vi "Redraw full indicator.vi"(8 "error in (no error)":errorcluster, 11 "D_Datagrid in":refnum<class "D_Datagrid.lvclass">) -> (0 "error out":errorcluster, 3 "D_Datagrid out":refnum<class "D_Datagrid.lvclass">)   [LabVIEW 2023, in "D Datagrid Library.lvlib" / "D_Datagrid.lvclass"]
doc: "Redraws the control to show the current DataElements value. If \"Auto Update Indicator\" is True, this is called automatically when writing DataElements. Otherwise, you should call this manually when you want to update the indicator."
uses:
  D_Datagrid.lvclass
  C:/Program Files/National Instruments/LabVIEW 2023/vi.lib/QSI/QControls/QControl Classes/Control/Control.lvclass
  C:/Program Files/National Instruments/LabVIEW 2023/vi.lib/QSI/QControls/QControl Classes/Table/Table.lvclass
  D_Datagrid.lvclass/D_Datagrid.ctl
  DatagridElement/DatagridElement.lvclass/DatagridElement.ctl
  <vilib>/Utility/miscctls.llb/LVRowAndColumnTypeDef.ctl
  DatagridElement/Read Cell font.vi
  DatagridElement/Read Text Alpha.vi
  DatagridElement/Read Enabled state.vi
  Read DataElements.vi
  <vilib>/Utility/colorconv.llb/Color to RGB.vi
  <vilib>/Utility/colorconv.llb/RGB to Color.vi
  DatagridElement/DatagridElement.lvclass
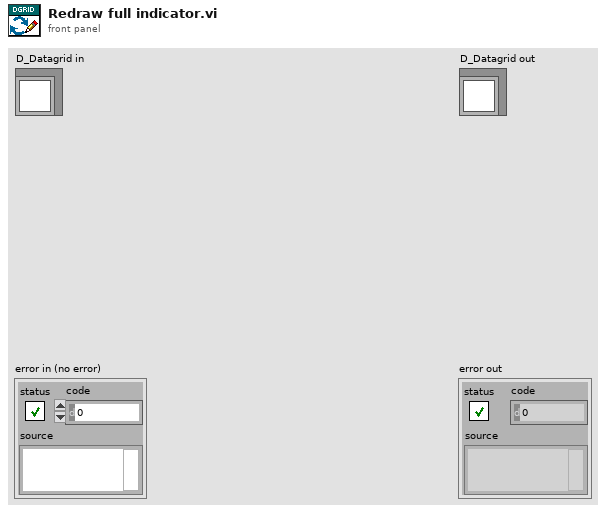
[diagram p1: front panel]
types:
  T1 = typedef "LVFontTypeDef.ctl" = cluster{"Font Name":string, "Size":u16, "Bold":bool, "Italic":bool, "Underline":bool, "Strikeout":bool, "Color":u32}
  T2 = enum8{"Enabled", "Disabled", "Disabled and Grayed Out"}
  T3 = cluster{"Accessors:Cell font":T1, "Accessors:Text Alpha":dbl, "Accessors:Enabled state":enum8{"Enabled", "Disabled", "Disabled and Grayed Out"}, i32, i32}
  T4 = typedef "LVRowAndColumnTypeDef.ctl" = cluster{"Row":i32, "Column":i32}
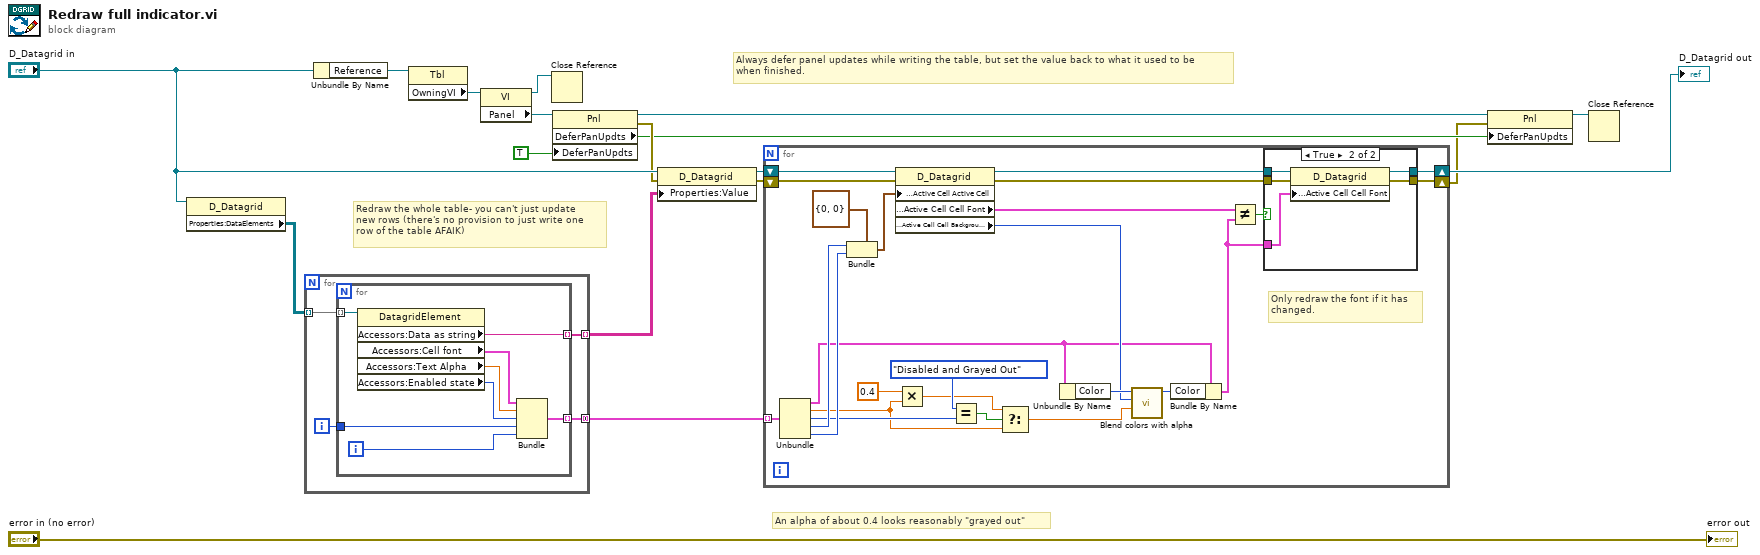
[diagram p0: block diagram]
diagram:
  # "An alpha of about 0.4 looks reasonably \"grayed out\""
  # "Redraw the whole table- you can't just update\nnew rows (there's no provision to just write one\nrow of the table AFAIK)"
  # "Always defer panel updates while writing the table, but set the value back to what it used to be\nwhen finished."
  n1 = property class="D_Datagrid"(reference="D_Datagrid in") -> ("Properties:DataElements"=w3:refnum<class "DatagridElement.lvclass">[][])  [unwired: 1 in, 2 out]
  n2 = for {
    tunnel: w3 -> [w22] mode=indexing
    tunnel: [w21] -> w15 mode=indexing
    tunnel: [w19] -> w13 mode=concatenating
    i -> [w20]
    n3 = for {
      tunnel: w22 -> [w30] mode=indexing
      tunnel: [w29] -> w21 mode=indexing
      tunnel: w20 -> [w28]
      tunnel: [w26] -> w19 mode=indexing
      i -> [w27]
      n4 = property class="DatagridElement"(reference=w30) -> ("Accessors:Data as string"=w29:string, "Accessors:Cell font"=w24:T1, "Accessors:Text Alpha"=w23:dbl, "Accessors:Enabled state"=w25:T2)  [unwired: 1 in, 2 out]
      n5 = Bundle("Accessors:Cell font"=w24, "Accessors:Text Alpha"=w23, "Accessors:Enabled state"=w25, w28, w27) -> (w26:T3)  [unwired: 1 in]
    }
  }
  n6 = Unbundle By Name("D_Datagrid in") -> ("Reference"=w12:refnum<vi>)
  n7 = property class="Tbl"(reference=w12) -> ("OwningVI"=w11:refnum<vi>)  [unwired: 1 in, 2 out]
  n8 = property class="VI"(reference=w11) -> (reference out=w9:refnum<vi>, "Panel"=w5:refnum<vi>)  [unwired: 1 in, 1 out]
  n9 = Close Reference(reference=w9) -> ()  [unwired: 1 in, 1 out]
  n10 = property class="Pnl"(reference=w5, "DeferPanUpdts"=TRUE ("Defer Panel Updates")) -> (reference out=w8:refnum<vi>, error out=w10:errorcluster, "DeferPanUpdts"=w4:bool)  [unwired: 1 in]
  n11 = property class="D_Datagrid"(reference="D_Datagrid in", error in=w10, "Properties:Value"=w15) -> (reference out=w14:refnum<class "D_Datagrid.lvclass">, error out=w2:errorcluster)
  n12 = for {
    shift-right: [w49] -> w16
    shift-left: w14 -> [w55]
    tunnel: w13 -> [w54] mode=indexing
    shift-right: [w44] -> w1
    shift-left: w2 -> [w46]
    # "Only redraw the font if it has\nchanged."
    n13 = Unbundle(w54) -> ("Accessors:Cell font"=w33:T1, "Accessors:Text Alpha"=w37:dbl, "Accessors:Enabled state"=w39:T2, w43:i32, w42:i32)
    n14 = Bundle(cluster=T4 {"Row"=0, "Column"=0} ("Active Cell:Active Cell"), "Row"=w43, "Column"=w42) -> (w51:T4)
    n15 = property class="D_Datagrid"(reference=w55, error in=w46, "Properties:Active Cell Active Cell"=w51) -> (reference out=w50:refnum<class "D_Datagrid.lvclass">, error out=w45:errorcluster, "Properties:Active Cell Cell Font"=w48:T1, "Properties:Active Cell Cell Background Color"=w35:u32)
    n16 = Multiply(x=0.4 ("y"), y=w37) -> (x*y=w38:dbl)
    n17 = Equal?(x=T2."Disabled and Grayed Out" ("Accessors:Enabled state"), y=w39) -> (x = y?=w40:bool)
    n18 = Select(t=w38, s=w40, f=w37) -> (s? t:f=w34:dbl)
    n19 = Unbundle By Name(w33) -> ("Color"=w36:u32)
    n20 = call "Blend colors with alpha.vi"("Top alpha"=w34, "Bottom color"=w35, "Top color"=w36) -> ("Result color"=w32:u32)  [unwired: 7 in, 1 out]
    n21 = Bundle By Name(cluster=w33, "Color"=w32) -> (w31:T1)
    n22 = Not Equal?(x=w48, y=w31) -> (x != y?=w47:bool)
    n23 = case shown="True" w47 {
      tunnel: w50 -> [w57 w62]
      tunnel: [w57 w61] -> w49
      tunnel: w45 -> [w56 w60]
      tunnel: [w56 w59] -> w44
      tunnel: w31 -> [_ w58]
      frame False {
      }
      frame True {
        n24 = property class="D_Datagrid"(reference=w62, error in=w60, "Properties:Active Cell Cell Font"=w58) -> (reference out=w61:refnum<class "D_Datagrid.lvclass">, error out=w59:errorcluster)
      }
    }
  }
  "D_Datagrid out" <- w16
  n25 = property class="Pnl"(reference=w8, error in=w1, "DeferPanUpdts"=w4) -> (reference out=w7:refnum<vi>)  [unwired: 1 out]
  n26 = Close Reference(reference=w7) -> ()  [unwired: 1 in, 1 out]
  "error out" <- "error in (no error)"
